vi "Get Type.vi"(8 "error in":errorcluster, 11 "CANopen Message in":refnum<class "CANopen Message.lvclass">) -> (0 "error out":errorcluster, 2 "Msg-Type":T1, 3 "CANopen Message out":refnum<class "CANopen Message.lvclass">)   [LabVIEW 2024, in "CANopen Master.lvlib" / "CANopen Message.lvclass"]
uses:
  CANopen Message.lvclass
  CANopen 2/Msg-Type.ctl
  CANopen Message.lvclass/CANopen Message.ctl
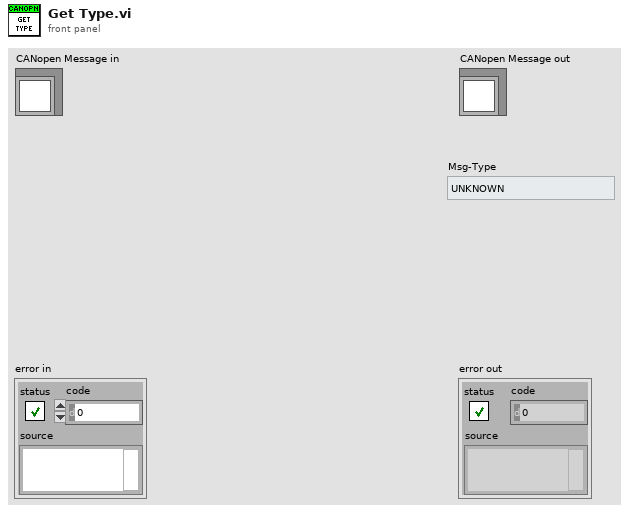
[diagram p1: front panel]
types:
  T1 = typedef "Msg-Type.ctl" = enum16{"UNKNOWN", "Initiate Download Request", "Initiate Upload Response", "Initiate Download Response", "Heartbeat"}
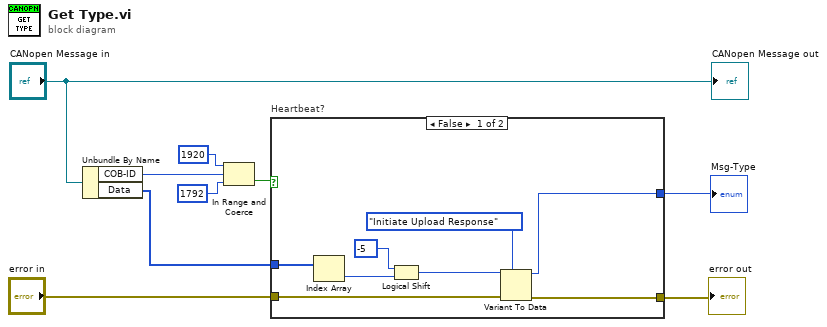
[diagram p0: block diagram]
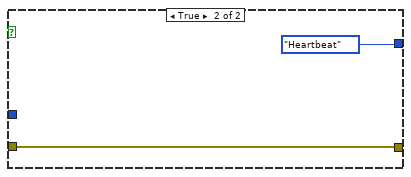
[diagram p2: hidden frame]
diagram:
  n1 = Unbundle By Name("CANopen Message in") -> ("COB-ID"=w6:u32, "Data"=w4:u8[])
  n2 = In Range and Coerce(upper limit=u32 1920 ("x"), x=w6, lower limit=u32 1792 ("x")) -> (In Range?=w5:bool)  [unwired: 1 out]
  n3 = case "Heartbeat?" shown="False" w5 {
    tunnel: w4 -> [w17 _]
    tunnel: [w10 Msg-Type."Heartbeat" ("Msg-Type")] -> w3
    tunnel: "error in" -> [w12 w18]
    tunnel: [w11 w18] -> w1
    frame False {
      n4 = Index Array(array=w17) -> (element=w15:u8)  [unwired: 1 in]
      n5 = Logical Shift(y=-5 ("x"), x=w15) -> (x << y=w13:u8)
      n6 = Variant To Data(error in=w12, type=Msg-Type."Initiate Upload Response" ("Msg-Type"), Variant=w13) -> (data=w10:T1, error out=w11:errorcluster)
    }
    frame True {
    }
  }
  "error out" <- w1
  "Msg-Type" <- w3
  "CANopen Message out" <- "CANopen Message in"
